vi "LabVIEWArduino2SLIDER.vi"() -> ()   [LabVIEW 2020]
uses:
  <vilib>/Instr/_visa.llb/VISA Configure Serial Port (Instr).vi
panel:
  in  "stop 2":bool
  in  "Slide":u8(slide) scale=0.0..65.0
  out "match substring":string
  in  "termination char\n(0xA = '\\n' = LF)":u8=10 format="%.0x"
  out "Waveform Graph":dbl[](graph)
  in  "VISA resource name":refnum<visa-resource-name>="COM3"
  in  "data bits (8)":u16=8 min=5 max=8 step=1
  in  "stop bits (10: 1 bit)":u16(ring)=10 items=["1.0"=10, "1.5"=15, "2.0"=20]
  in  "flow control (0:none)":u16(ring) items=["None", "XON/XOFF", "RTS/CTS", "XON/XOFF & RTS/CTS", "DTR/DSR", "XON/XOFF & DTR/DSR"]
  in  "parity (0:none)":enum16{"None", "Odd", "Even", "Mark", "Space"}(ring)
  out "TempArray":dbl[](array[numeric]) caption="Temperature Array"
  out "CurTemp":dbl caption="Current Temperature\n(Celsius)"
  in  "stop":bool
  in  "Emergency Stop!":bool
  in  "Decellerate":bool
  in  "Motor Control Duino":refnum<visa-resource-name>
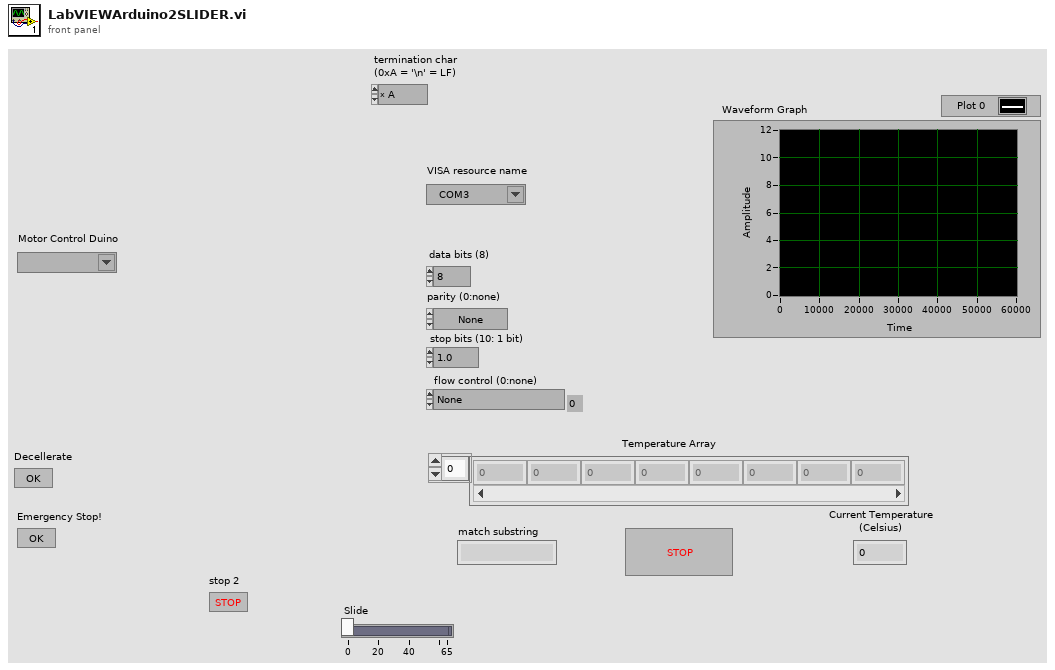
[diagram p1: front panel]
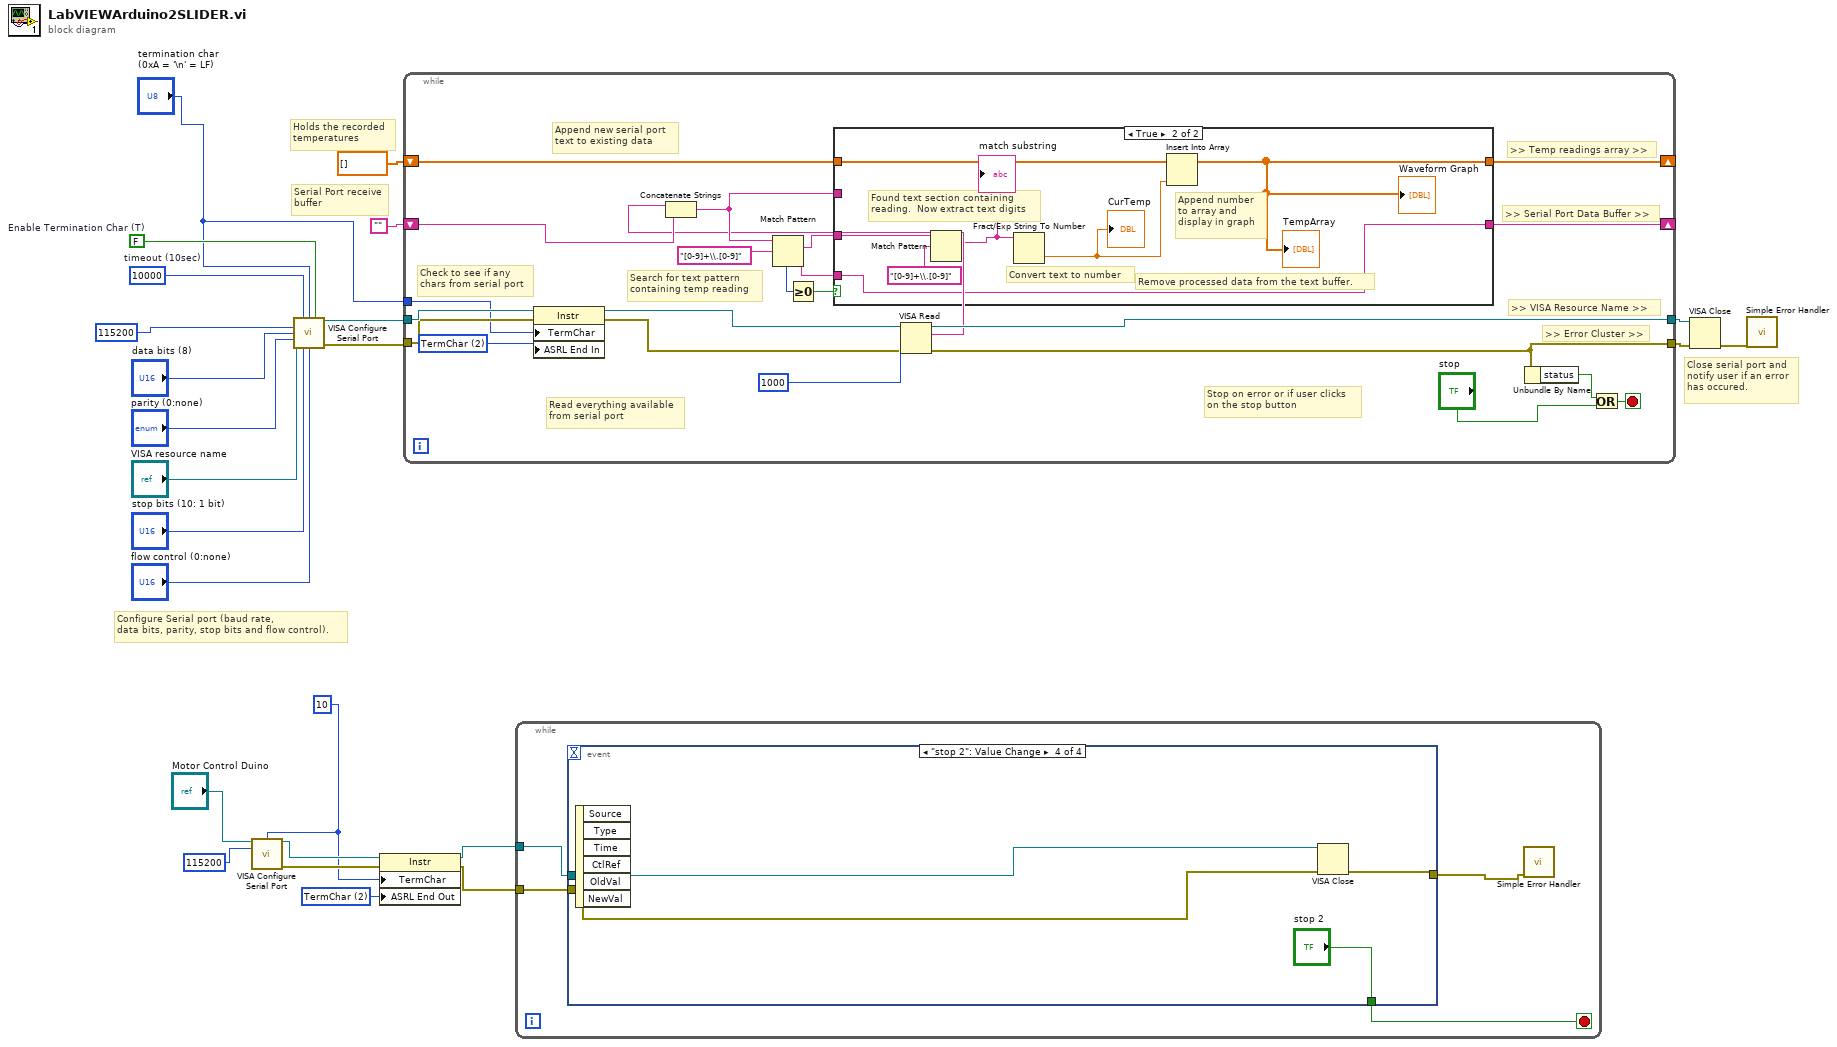
[diagram p0: block diagram]
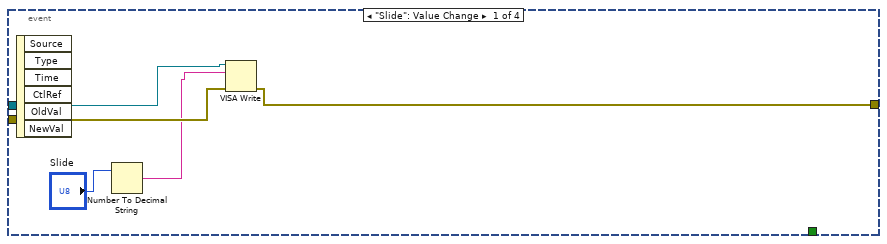
[diagram p3: hidden frame]
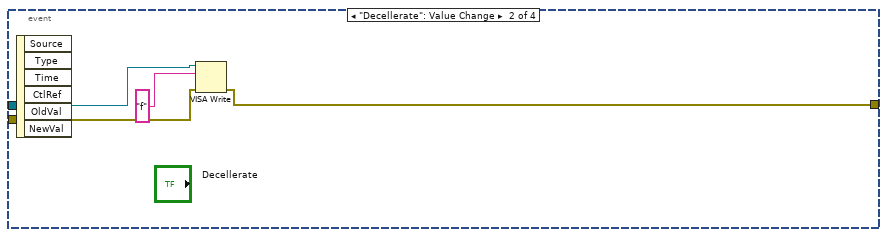
[diagram p4: hidden frame]
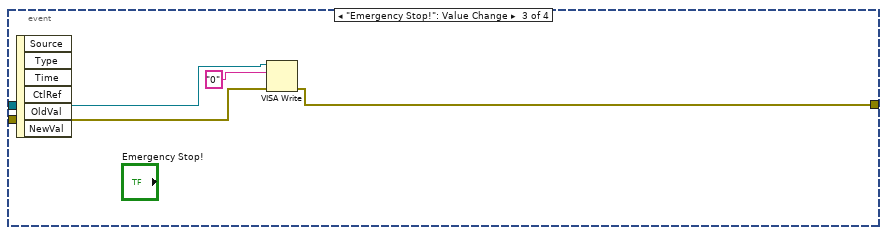
[diagram p5: hidden frame]
diagram:
  w1 = u16 2 items=["None", "Last Bit", "TermChar", "Break"] ("Serial Settings:End Mode for Writes")
  w2 = u8 10 ("termination char\n(0xA = '\\n' = LF)")
  w18 = FALSE  # Enable Termination Char (T)
  w19 = u32 10000  # timeout (10sec)
  # "Close serial port and\nnotify user if an error\nhas occured."
  # "Serial Port receive\nbuffer"
  # "Holds the recorded\ntemperatures"
  # "Configure Serial port (baud rate,\ndata bits, parity, stop bits and flow control)."
  n1 = call-poly "VISA Configure Serial Port"("VISA resource name"="Motor Control Duino", "termination char\n(0xA = '\\n' = LF)"=w2, "baud rate (9600)"=u32 115200) -> ("VISA resource name out"=w6:refnum<visa-resource-name>, "error out"=w3:errorcluster)  [unwired: 11 in]
  n2 = call-poly "VISA Configure Serial Port"("VISA resource name"="VISA resource name", "timeout (10sec)"=w19, "termination char\n(0xA = '\\n' = LF)"="termination char\n(0xA = '\\n' = LF)", "Enable Termination\nChar (T)"=w18, "baud rate (9600)"=u32 115200, "data bits (8)"="data bits (8)", "parity (0:none)"="parity (0:none)", "stop bits (10: 1 bit)"="stop bits (10: 1 bit)", "flow control (0:none)"="flow control (0:none)") -> ("VISA resource name out"=w8:refnum<visa-resource-name>, "error out"=w7:errorcluster)  [unwired: 5 in]
  n3 = property class="Instr"(reference=w6, error in=w3, "TermChar"=w2, "ASRL End Out"=w1) -> (reference out=w5:refnum<visa-resource-name>, error out=w4:errorcluster)
  n4 = while {
    tunnel: [w45] -> w22
    tunnel: [w47] -> w21
    shift-right: [w40] -> _
    shift-left: "" -> [w46]
    tunnel: w8 -> [w31]
    tunnel: w7 -> [w30]
    shift-right: [w42] -> _
    shift-left: dbl[] [] -> [w41]
    tunnel: "termination char\n(0xA = '\\n' = LF)" -> [w27]
    stop <- w44 stop-if-true
    w26 = u16 2 items=["None", "Last Bit", "TermChar"] ("Serial Settings:End Mode for Reads")
    # "Search for text pattern\ncontaining temp reading"
    # "Append new serial port\ntext to existing data"
    # "Read everything available\nfrom serial port"
    # "Stop on error or if user clicks \non the stop button"
    # ">> Error Cluster >>"
    # ">> VISA Resource Name >>"
    # ">> Temp readings array >>"
    # ">> Serial Port Data Buffer >>"
    # "Check to see if any\nchars from serial port"
    n5 = property class="Instr"(reference=w31, error in=w30, "TermChar"=w27, "ASRL End In"=w26) -> (reference out=w29:refnum<visa-resource-name>, error out=w28:errorcluster)
    n6 = VISA Read(VISA resource name=w29, byte count=u32 1000, error in (no error)=w28) -> (VISA resource name out=w47:refnum<visa-resource-name>, read buffer=w33:string, error out=w45:errorcluster)  [unwired: 1 out]
    n7 = Concatenate Strings(w33, w46) -> (w34:string)
    n8 = Match Pattern(string=w34, regular expression="[0-9]+\\.[0-9]") -> (match substring=w36:string, after substring=w35:string, offset past match=w38:i32)  [unwired: 1 in, 1 out]
    n9 = Greater Or Equal To 0?(x=w38) -> (x >= 0?=w37:bool)
    n10 = case shown="True" w37 {
      tunnel: w36 -> [_ w55]
      tunnel: w35 -> [_ w56]
      tunnel: w34 -> [w49 _]
      tunnel: [w49 w56] -> w40
      tunnel: [w48 w50] -> w42
      tunnel: w41 -> [w48 w53]
      frame False {
        # "Did not find text pattern in the buffer.  Try again in the next loop after new data \nhas been received."
      }
      frame True {
        # "Remove processed data from the text buffer."
        # "Append number\nto array and\ndisplay in graph"
        # "Convert text to number"
        # "Found text section containing \nreading.  Now extract text digits"
        n11 = Match Pattern(string=w55, regular expression="[0-9]+\\.[0-9]") -> (match substring=w54:string)  [unwired: 1 in, 3 out]
        "match substring" <- w54
        n12 = Fract/Exp String To Number(string=w54) -> (number=w51:dbl)  [unwired: 3 in, 1 out]
        "CurTemp" <- w51
        n13 = Insert Into Array(array=w53, new element=w51) -> (w50:dbl[])  [unwired: 1 in]
        "TempArray" <- w50
        "Waveform Graph" <- w50
      }
    }
    n14 = Unbundle By Name(w45) -> ("status"=w43:bool)
    n15 = Or(x=w43, y="stop") -> (x .or. y?=w44:bool)
  }
  n16 = while {
    tunnel: w5 -> [w60]
    tunnel: w4 -> [w59]
    stop <- w57 stop-if-true
    n17 = event shown="[3] \"stop 2\": Value Change" {
      selector: _ -> [_ _ _ _]
      dyn-events: _ -> [_ _ _ _]
      timeout: _ -> [_ _ _ _]
      tunnel: [w65 w69 w73 w77] -> w58
      tunnel: w60 -> [w64 w67 w71 w76]
      tunnel: w59 -> [w63 w66 w70 w75]
      tunnel: [_ _ _ "stop 2"] -> w57
      event "Slide": Value Change {
        n18 = event-data() -> ()  [unwired: 1 in, 6 out]
        n19 = Number To Decimal String(number="Slide") -> (decimal integer string=w62:string)  [unwired: 1 in]
        n20 = VISA Write(VISA resource name=w64, write buffer=w62, error in (no error)=w63) -> (error out=w65:errorcluster)  [unwired: 2 out]
      }
      event "Decellerate": Value Change {
        n21 = event-data() -> ()  [unwired: 1 in, 6 out]
        n22 = VISA Write(VISA resource name=w67, write buffer="f", error in (no error)=w66) -> (error out=w69:errorcluster)  [unwired: 2 out]
      }
      event "Emergency Stop!": Value Change {
        n23 = event-data() -> ()  [unwired: 1 in, 6 out]
        n24 = VISA Write(VISA resource name=w71, write buffer="0", error in (no error)=w70) -> (error out=w73:errorcluster)  [unwired: 2 out]
      }
      event "stop 2": Value Change {
        n25 = event-data() -> ()  [unwired: 1 in, 6 out]
        n26 = VISA Close(VISA resource name=w76, error in (no error)=w75) -> (error out=w77:errorcluster)
      }
    }
    n27 = call <vilib>:"Simple Error Handler.vi"("error in (no error)"=w58) -> ()  [unwired: 4 in, 5 out]
  }
  n28 = VISA Close(VISA resource name=w21, error in (no error)=w22) -> (error out=w20:errorcluster)
  n29 = call <vilib>:"Simple Error Handler.vi"("error in (no error)"=w20) -> ()  [unwired: 4 in, 5 out]
